vi "AVS_Get_T.vi"(9 "Sensor Calib":i8, 10 "AVS Channel":i8, 11 "Wait for channel (s)":i8) -> (2 "Resistance reading":dbl format="%.2f", 3 "T (K)":dbl=0.00957168277075326 format="%^.3e")   [LabVIEW 2018]
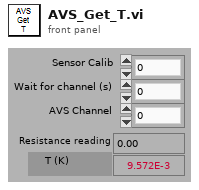
[diagram p1: front panel]
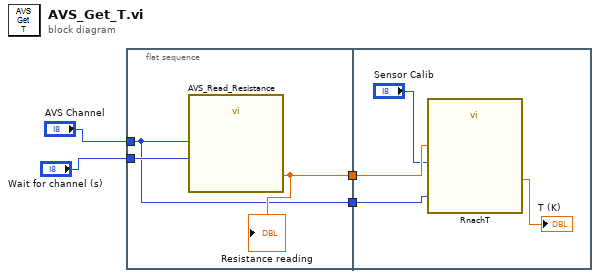
[diagram p0: block diagram]
diagram:
  n1 = flat-sequence {
    tunnel: [w7] -> w4
    tunnel: "AVS Channel" -> [w5]
    tunnel: "Wait for channel (s)" -> [w6]
    tunnel: [w5] -> w1
    tunnel: w4 -> [w10]
    tunnel: w1 -> [w8]
    frame #0 {
      n2 = call "AVS_Read_Resistance.vi"("Wait for channel (s)"=w6, "AVS Channel"=w5) -> ("AVS Resistance reading"=w7:dbl)  [unwired: 9 in]
      "Resistance reading" <- w7
    }
    frame #1 {
      n3 = call "RnachT.vi"("AVS Channel"=w8, "R"=w10, "Sensor Cal#"="Sensor Calib") -> ("T (K)"=→"T (K)":dbl)
    }
  }
